vi "errors.vi"(0 "errors":T1=enum."noDevices", 7 "dialog? (T)":bool=TRUE, 9 "transmit? (T)":bool=TRUE, 12 "supp_text":string[](array[string])) -> (15 "error out":errorcluster)   [LabVIEW 2012]
doc: "Traps and handles errors commonly seen during Performax hardware communication.\n\nProduced By:\n\nChristopher Lemieux\nKod Integrations, LLC\n4835 Marianne Drive\nMount Airy, MD 21771\nhttp://www.kodintegrations.com\nemail: clemieux@kodintegrations.com\nphone: (240) 687-1288"
uses:
  controls/errors_actions.ctl
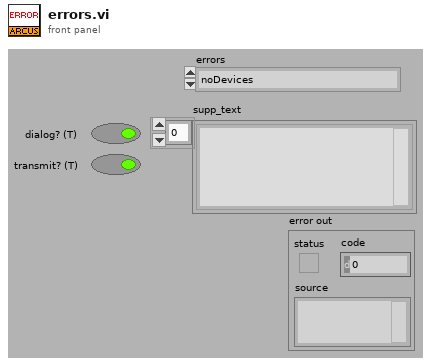
[diagram p1: front panel]
types:
  T1 = typedef "errors_actions.ctl" = enum16{"clearBuff", "closeRef", "noDeviceInfo", "noDevices", "openRef", "sendReceive", "setTimeouts", "unknown"}
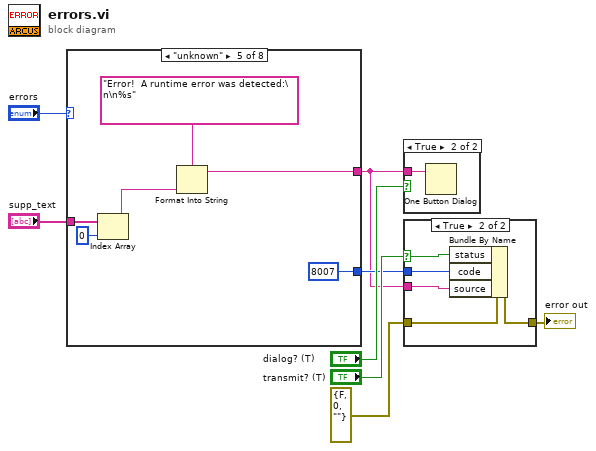
[diagram p0: block diagram]
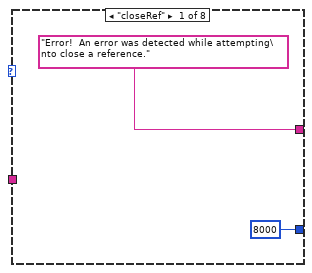
[diagram p4: hidden frame]
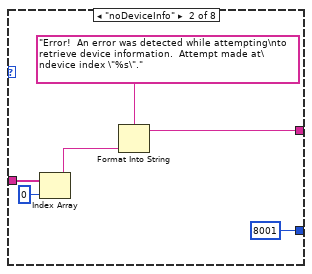
[diagram p5: hidden frame]
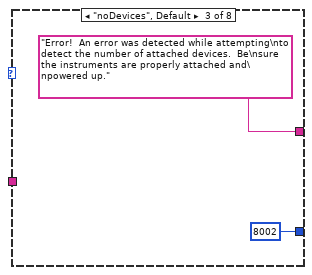
[diagram p6: hidden frame]
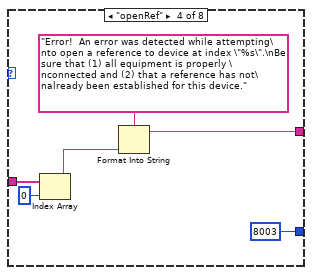
[diagram p7: hidden frame]
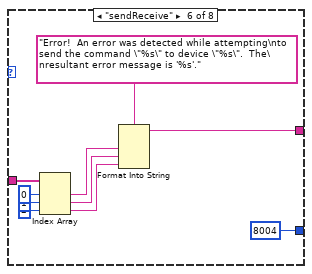
[diagram p8: hidden frame]
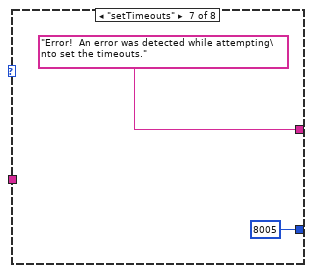
[diagram p9: hidden frame]
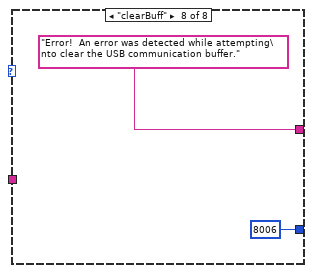
[diagram p10: hidden frame]
diagram:
  n1 = case shown="\"unknown\"" "errors" {
    tunnel: ["Error!  An error was detected while attempting\nto close a reference." w12 "Error!  An error was detected while attempting\nto detect the number of attached devices.  Be\nsure the instruments are properly attached and\npowered up." w20 w26 w36 "Error!  An error was detected while attempting\nto set the timeouts." "Error!  An error was detected while attempting\nto clear the USB communication buffer."] -> w2
    tunnel: [8000 8001 8002 8003 8007 8004 8005 8006] -> w5
    tunnel: "supp_text" -> [_ w15 _ w23 w29 w39 _ _]
    frame "closeRef" {
    }
    frame "noDeviceInfo" {
      n2 = Index Array(array=w15, index=0) -> (element=w13:string)
      n3 = Format Into String(format string="Error!  An error was detected while attempting\nto retrieve device information.  Attempt made at\ndevice index \"%s\".", w13) -> (resulting string=w12:string)  [unwired: 2 in, 1 out]
    }
    frame "noDevices", Default {
    }
    frame "openRef" {
      n4 = Index Array(array=w23, index=0) -> (element=w21:string)
      n5 = Format Into String(format string="Error!  An error was detected while attempting\nto open a reference to device at index \"%s\".\nBe sure that (1) all equipment is properly \nconnected and (2) that a reference has not\nalready been established for this device.", w21) -> (resulting string=w20:string)  [unwired: 2 in, 1 out]
    }
    frame "unknown" {
      n6 = Index Array(array=w29, index=0) -> (element=w27:string)
      n7 = Format Into String(format string="Error!  A runtime error was detected:\n\n%s", w27) -> (resulting string=w26:string)  [unwired: 2 in, 1 out]
    }
    frame "sendReceive" {
      n8 = Index Array(array=w39, index #1=0 ("index"), index #2=1 ("index"), index #3=2 ("index")) -> (element #1=w37:string, element #2=w33:string, element #3=w31:string)
      n9 = Format Into String(format string="Error!  An error was detected while attempting\nto send the command \"%s\" to device \"%s\".  The\nresultant error message is '%s'.", w37, w33, w31) -> (resulting string=w36:string)  [unwired: 2 in, 1 out]
    }
    frame "setTimeouts" {
    }
    frame "clearBuff" {
    }
  }
  n10 = case shown="True" "dialog? (T)" {
    tunnel: w2 -> [_ w45]
    frame False {
    }
    frame True {
      n11 = One Button Dialog(message=w45) -> ()  [unwired: 1 in, 1 out]
    }
  }
  n12 = case shown="True" "transmit? (T)" {
    selector: "transmit? (T)" -> [_ w48]
    tunnel: errorcluster {"status"=FALSE, "code"=0, "source"=""} ("error out") -> [w46 w51]
    tunnel: w5 -> [_ w50]
    tunnel: w2 -> [_ w49]
    tunnel: [w46 w47] -> w4
    frame False {
    }
    frame True {
      n13 = Bundle By Name(cluster=w51, "status"=w48, "code"=w50, "source"=w49) -> (w47:errorcluster)
    }
  }
  "error out" <- w4
